vi "setwavelength.vi"(5 "Dup Visa Session":refnum<visa-resource-name>, 6 "Set Wavelength":string="275", 7 "error in (no error)":errorcluster) -> (0 "dup Visa Session":refnum<visa-resource-name>, 3 "error out":errorcluster)   [LabVIEW 2012]
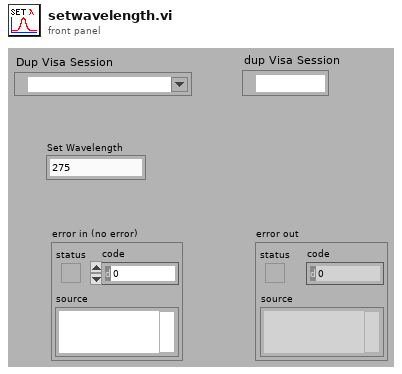
[diagram p1: front panel]
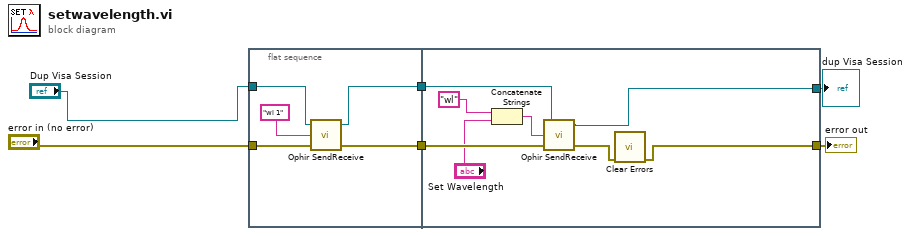
[diagram p0: block diagram]
diagram:
  n1 = flat-sequence {
    tunnel: [w10] -> w5
    tunnel: "error in (no error)" -> [w9]
    tunnel: "Dup Visa Session" -> [w8]
    tunnel: [w7] -> w4
    tunnel: [w12] -> w6
    tunnel: [w14] -> w3
    tunnel: w5 -> [w19]
    tunnel: w4 -> [w18]
    frame #0 {
      n2 = call "Ophir SendReceive.vi"("error in (no error)"=w9, "Command"="wi 1", "Visa Session"=w8) -> ("error out"=w10:errorcluster, "dup Visa Session"=w7:refnum<visa-resource-name>)  [unwired: 1 out]
    }
    frame #1 {
      n3 = Concatenate Strings("wl" ("Command"), "Set Wavelength") -> (w15:string)
      n4 = call "Ophir SendReceive.vi"("error in (no error)"=w19, "Command"=w15, "Visa Session"=w18) -> ("error out"=w13:errorcluster, "dup Visa Session"=w14:refnum<visa-resource-name>)  [unwired: 1 out]
      n5 = call <vilib>:"Clear Errors.vi"("error in (no error)"=w13) -> ("error out"=w12:errorcluster)  [unwired: 6 in]
    }
  }
  "error out" <- w6
  "dup Visa Session" <- w3
